vi "Scalar Polynomial Evaluation (CDB).vi"(2 "P(x)":cdb[](array[numeric]) format="%#.2f", 3 "a":cdb) -> (0 "error":i32, 1 "P(a)":cdb)   [LabVIEW 2020, in "NI_AALPro.lvlib"]
doc: "Evaluates the polynomial <B>P(x)</B> with a single value or multiple values. The data types you wire to the <B>a</B> and <B>P(x)</B> inputs determine the polymorphic instance to use."
uses:
  <vilib>/Analysis/NI_AALPro.lvlib
  <vilib>/Analysis/polynomials.llb/Remove Zero Coefficients (CDB).vi
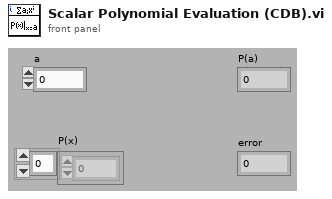
[diagram p1: front panel]
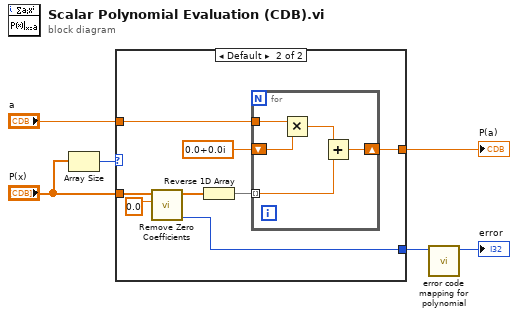
[diagram p0: block diagram]
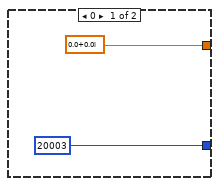
[diagram p2: hidden frame]
diagram:
  n1 = Array Size(array="P(x)") -> (size(s)=w6:i32)
  n2 = case shown="Default" w6 {
    tunnel: "a" -> [_ w14]
    tunnel: [cdb 0.0+0.0i w13] -> w4
    tunnel: [20003 ("empty array") w9] -> w2
    tunnel: "P(x)" -> [_ w11]
    frame 0 {
    }
    frame Default {
      n3 = call-poly <vilib>:"Remove Zero Coefficients.vi"("threshold"=0.0, "P(x) In"=w11) -> ("error"=w9:i32, "P(x) Out"=w10:cdb[])  [unwired: 7 in, 1 out]
      n4 = Reverse 1D Array(array=w10) -> (reversed array=w15:cdb[])
      n5 = for {
        shift-right: [w17] -> w13
        shift-left: cdb 0.0+0.0i -> [w20]
        tunnel: w14 -> [w21]
        tunnel: w15 -> [w19] mode=indexing
        n6 = Multiply(x=w21, y=w20) -> (x*y=w18:cdb)
        n7 = Add(x=w18, y=w19) -> (x+y=w17:cdb)
      }
    }
  }
  "P(a)" <- w4
  n8 = call <vilib>:"error code mapping for polynomial.vi"("error in"=w2) -> ("error out"=→"error":i32)  [unwired: 10 in]
